vi "Read Data_HoldingRegistors.vi"(8 "error in (no error)":errorcluster, 11 "Device in":refnum<class "DAQ_Device.lvclass">) -> (0 "error out":errorcluster, 2 "register values":dbl[](array[numeric]), 3 "Device out":refnum<class "DAQ_Device.lvclass">)   [LabVIEW 2023, in "DAQ_Device.lvclass"]
uses:
  DAQ_Device.lvclass
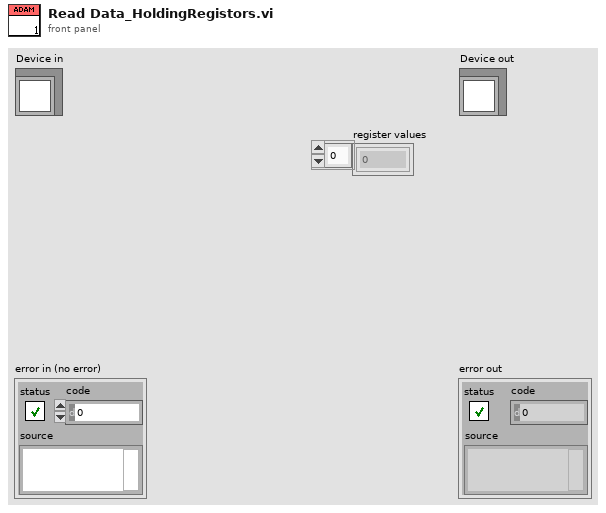
[diagram p1: front panel]
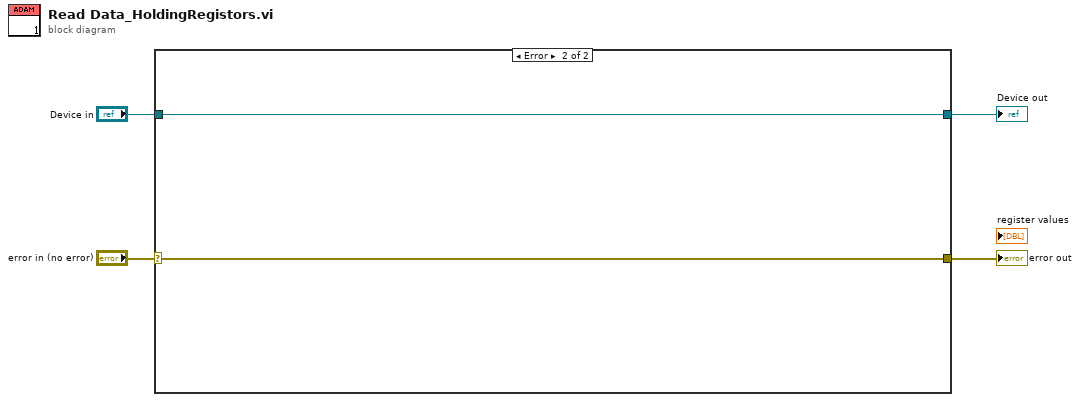
[diagram p0: block diagram]
diagram:
  n1 = case shown="Error" "error in (no error)" {
    selector: "error in (no error)" -> [w6 w8]
    tunnel: [w6 w8] -> w3
    tunnel: [w5 w7] -> w1
    tunnel: "Device in" -> [w5 w7]
    frame No Error {
    }
    frame Error {
    }
  }
  "error out" <- w3
  "Device out" <- w1
